vi "EditVIPBLVVersion.vi"(7 "labview version":string, 8 "error in":errorcluster, 11 "path to vipb file":path) -> (0 "error out":errorcluster)   [LabVIEW 2019]
uses:
  <vilib>/regexp/Match Regular Expression.xnode
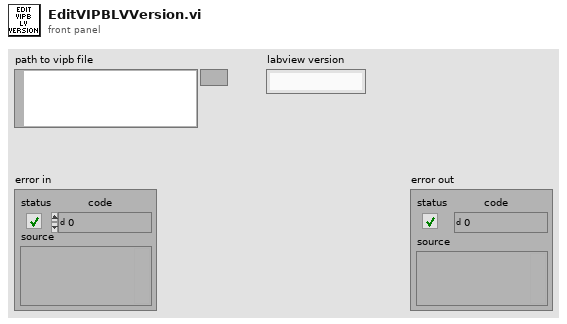
[diagram p1: front panel]
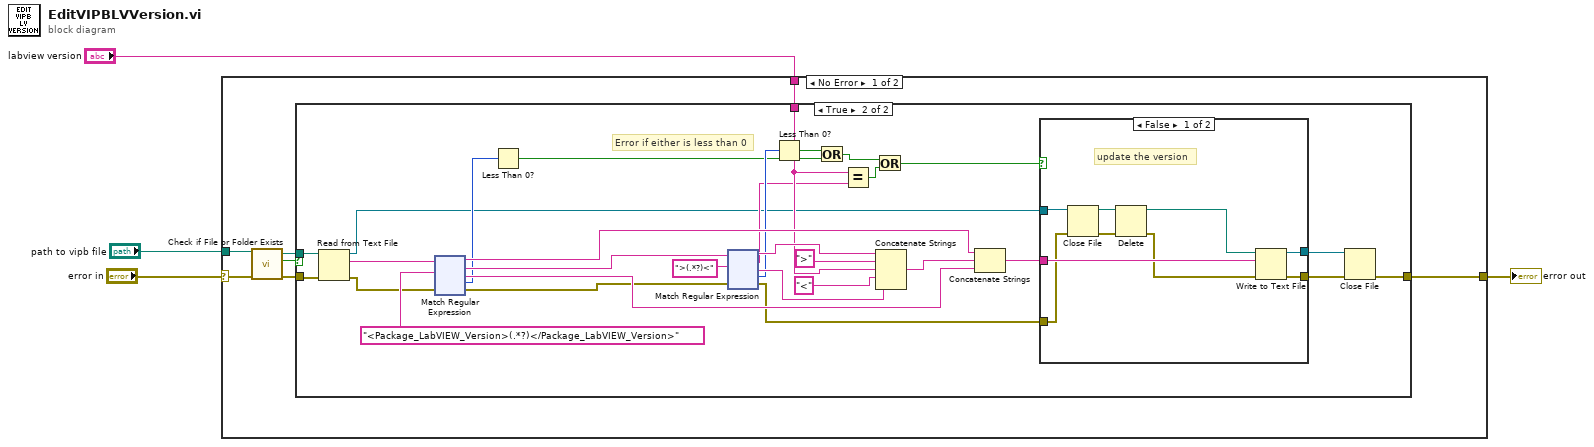
[diagram p0: block diagram]
diagram:
  n1 = case shown="No Error" "error in" {
    selector: "error in" -> [w9 w282]
    tunnel: "labview version" -> [w11 _]
    tunnel: "path to vipb file" -> [w10 _]
    tunnel: [w5 w282] -> w1
    frame No Error {
      n2 = call <vilib>:"Check if File or Folder Exists.vi"("error in (no error)"=w9, "path"=w10) -> ("error out"=w7:errorcluster, "file or folder exists?"=w8:bool, "dup path"=w6:path)  [unwired: 7 in]
      n3 = case shown="True" w8 {
        tunnel: w11 -> [_ w25]
        tunnel: w7 -> [w12 w31]
        tunnel: w6 -> [_ w32]
        tunnel: [w12 w13] -> w5
        frame False {
        }
        frame True {
          # "Error if either is less than 0"
          n4 = Read from Text File(file (use dialog)=w32, error in=w31) -> (refnum out=w19:refnum<file>, text=w30:string, error out=w17:errorcluster)  [unwired: 2 in, 1 out]
          n5 = xnode "Match Regular Expression"("input string"=w30, "regular expression"="<Package_LabVIEW_Version>(.*?)</Package_LabVIEW_Version>", "error in"=w17) -> ("before match"=w35:string, "whole match"=w41:string, "after match"=w33:string, "offset past match"=w29:i32, "error out"=w16:errorcluster)  [unwired: 3 in]
          n6 = Less Than 0?(x=w29) -> (x < 0?=w26:bool)
          n7 = xnode "Match Regular Expression"("input string"=w41, "regular expression"=">(.*?)<", "error in"=w16) -> ("before match"=w37:string, "whole match"=w24:string, "after match"=w36:string, "offset past match"=w28:i32, "error out"=w15:errorcluster)  [unwired: 3 in]
          n8 = Less Than 0?(x=w28) -> (x < 0?=w27:bool)
          n9 = Or(x=w27, y=w26) -> (x .or. y?=w22:bool)
          n10 = Equal?(x=w25, y=w24) -> (x = y?=w23:bool)
          n11 = Or(x=w22, y=w23) -> (x .or. y?=w21:bool)
          n12 = Concatenate Strings(w37, ">", w25, "<", w36) -> (w34:string)
          n13 = Concatenate Strings(w35, w34, w33) -> (w20:string)
          n14 = case shown="False" w21 {
            tunnel: w20 -> [w49 _]
            tunnel: w19 -> [w48 w53]
            tunnel: [w50 w53] -> w18
            tunnel: w15 -> [w47 w52]
            tunnel: [w51 w52] -> w14
            frame False {
              # "update the version"
              n15 = Close File(refnum=w48, error in=w47) -> (path=w45:path, error out=w46:errorcluster)
              n16 = Delete(path (use dialog)=w45, error in=w46) -> (deleted path=w43:path, error out=w44:errorcluster)  [unwired: 3 in, 1 out]
              n17 = Write to Text File(file (use dialog)=w43, text=w49, error in=w44) -> (refnum out=w50:refnum<file>, error out=w51:errorcluster)  [unwired: 1 in, 1 out]
            }
            frame True {
              # "Either an Error or file does not need editing"
            }
          }
          n18 = Close File(refnum=w18, error in=w14) -> (error out=w13:errorcluster)  [unwired: 1 out]
        }
      }
    }
    frame Error {
      # "If there is already an error, do not edit the file"
    }
  }
  "error out" <- w1
